vi "degreesToPot.vi"(9 "POT VALUE AT 80*":dbl=0.6, 10 "POT VALUE AT 50*":dbl=0.5, 11 "ANGLE(DEGREES)":dbl) -> (3 "POT VALUE (0-1)":dbl)   [LabVIEW 2012]
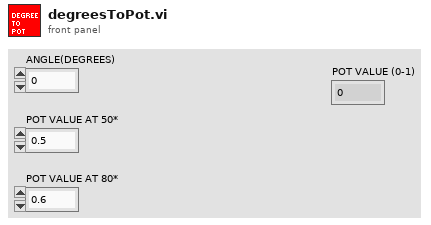
[diagram p1: front panel]
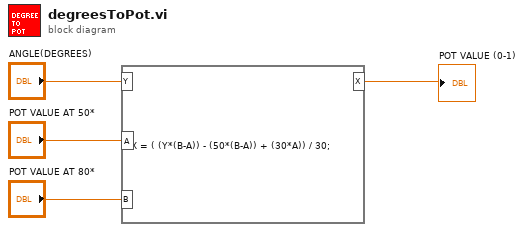
[diagram p0: block diagram]
diagram:
  n1 = formula code="X = ( (Y*(B-A)) - (50*(B-A)) + (30*A)) / 30;"("Y"="ANGLE(DEGREES)", "A"="POT VALUE AT 50*", "B"="POT VALUE AT 80*") -> ("X"=→"POT VALUE (0-1)":dbl)
